vi "final.vi"() -> ()   [LabVIEW 2018]
uses:
  <vilib>/imath/engines/lvmath2/RunTimeEngine/Managers/WorkSpace/UID Generator.vi
  <vilib>/imath/engines/lvmath2/RunTimeEngine/RunTimeType/NIMS_RunTimeType_From StrictType (excl LVString).vi
  <instcachedir>/0/NIMS_RunTimeType_From StrictType (excl LVString)_E7E34A65C99947108168652BAD14964D.lvgen/NIMS_RunTimeType_From StrictType (excl LVString)_E7E34A65C99947108168652BAD14964D_000.vi
  <vilib>/imath/engines/lvmath2/RunTimeEngine/LocalVariableDefStatement/MC_LocalVariableDefStatement_Display.vi
  <vilib>/imath/engines/lvmath2/RunTimeEngine/RangeToken/NIMS_Range_R2 - Integer.vi
  <instcachedir>/0/NIMS_Range_R2 - Integer_E35B921DECF84AADB7325A02D418BFCC.lvgen/NIMS_Range_R2 - Integer_E35B921DECF84AADB7325A02D418BFCC_000.vi
  <vilib>/imath/engines/lvmath2/RunTimeEngine/CommandStatement/MC_CommandStatement_break.vi
  <vilib>/imath/engines/lvmath2/RunTimeEngine/IndexRead/NIMS V(S).vi
  <instcachedir>/0/NIMS V(S)_0488751826AF41519A22953C041130DC.lvgen/NIMS V(S)_0488751826AF41519A22953C041130DC_000.vi
  <vilib>/imathl/engines/lvmath/Functions/Error Handling/Create Error.vi
  <vilib>/imath/engines/lvmath2/RunTimeEngine/Managers/SymbolTable/Clear UID.vi
  <vilib>/imath/engines/lvmath2/RunTimeEngine/NodeEndStatement/NIMS_NodeEndStatement_Output.vi
  <instcachedir>/0/NIMS_NodeEndStatement_Output_53EC0D466D134D7ABD903AC30B43404B.lvgen/NIMS_NodeEndStatement_Output_53EC0D466D134D7ABD903AC30B43404B_011.vi
  <vilib>/imath/engines/lvmath2/RunTimeEngine/ErrorHandling/NIMS_Finalize Error.vi
  <vilib>/imath/engines/lvmath2/RunTimeEngine/BuiltInFunctions/acos/NIMS_acos(C).vi
  <instcachedir>/0/NIMS_acos(C)_EB9F8BBCD4F84158BAE4AC9B979C42E8.lvgen/NIMS_acos(C)_EB9F8BBCD4F84158BAE4AC9B979C42E8_001.vi
  <instcachedir>/0/NIMS_NodeEndStatement_Output_53EC0D466D134D7ABD903AC30B43404B.lvgen/NIMS_NodeEndStatement_Output_53EC0D466D134D7ABD903AC30B43404B_001.vi
  <vilib>/imath/engines/lvmath2/RunTimeEngine/Managers/SymbolTable/NIMS_WorkSpace.lvlib
panel:
  in  "Position 2":cluster{"X":dbl, "Y":dbl, "Theta":dbl}
  out "idx":i32=10
  in  "Position":cluster{"X":dbl, "Y":dbl, "Theta":dbl}
  out "range Out":dbl[](array[numeric])
  out "Position (mm)":cluster{"X":dbl, "Y":dbl, "Theta":dbl}
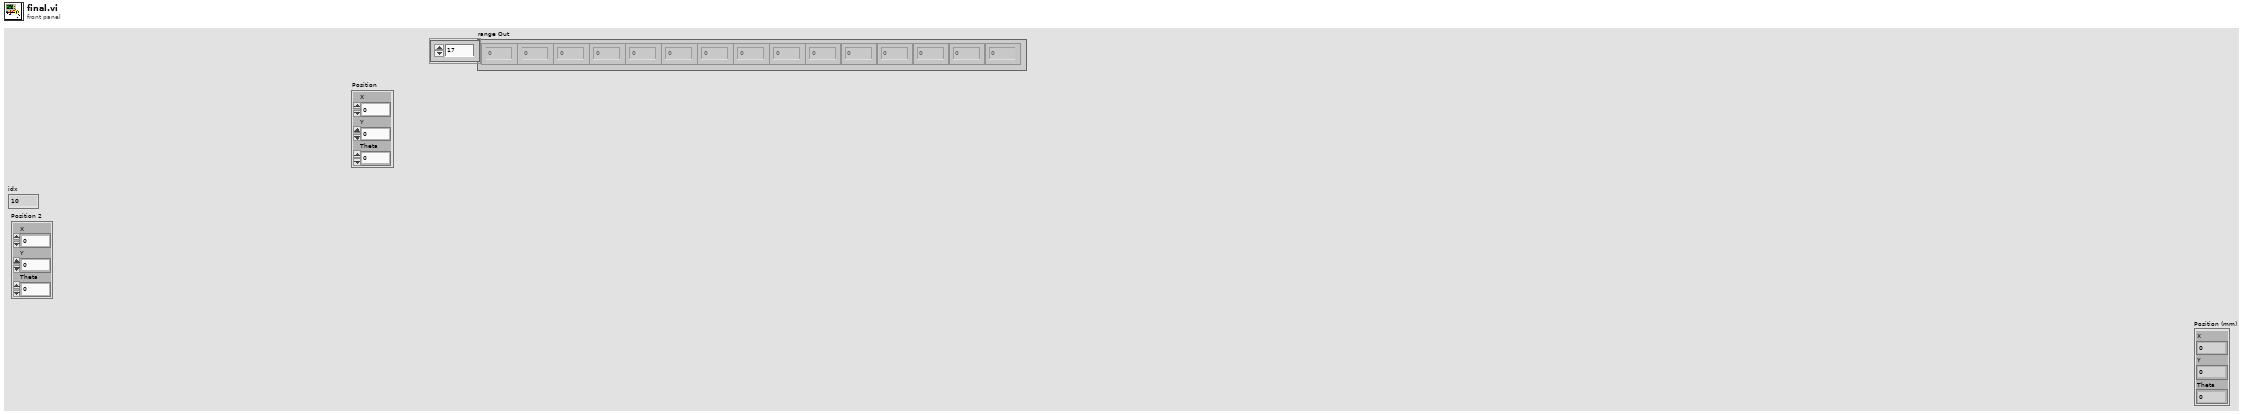
[diagram p1: front panel]
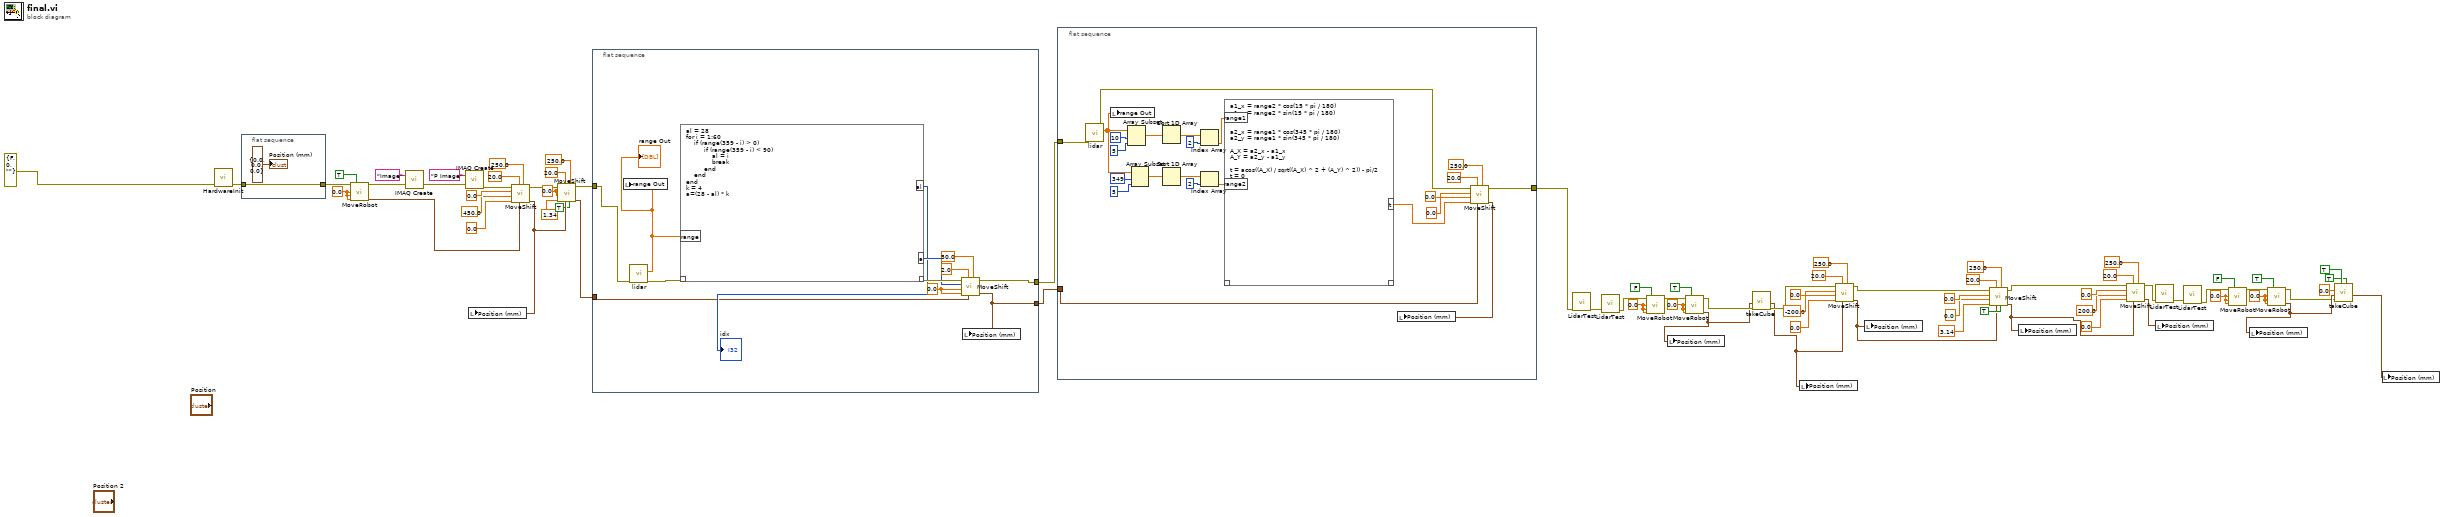
[diagram p0: block diagram]
diagram:
  w15 = 0.0 ("x (mm/s)")
  w12 = 0.0 ("x (mm/s)")
  w40 = 0.0 ("x (mm/s)")
  w43 = 0.0 ("x (mm/s)")
  w56 = 0.0 ("x shift")
  w74 = 0.0 ("x (mm/s)")
  n1 = call "HardwareInit.vi"("Error/Flow In"=errorcluster {"status"=FALSE, "code"=0, "source"=""}) -> ("error out"=w61:errorcluster)  [unwired: 10 in]
  n2 = flat-sequence {
    tunnel: w61 -> [w75]
    tunnel: [w75] -> w60
    frame #0 {
      "Position (mm)" <- cluster{"X":dbl, "Y":dbl, "Theta":dbl} {"X"=0.0, "Y"=0.0, "Theta"=0.0} ("Position (mm)")
    }
  }
  n3 = call "MoveRobot.vi"("Error/Flow In"=w60, "Reset"=TRUE, "x (mm/s)"=w74, "y (mm/s)"=w74, "theta (rad/s)"=w74) -> ("Error/Flow Out"=w72:errorcluster, "Position"=w62:cluster{"X":dbl, "Y":dbl, "Theta":dbl})  [unwired: 9 in]
  n4 = call "IMAQ Create"("Image Name"="Image", "error in (no error)"=w72) -> ("error out"=w70:errorcluster)  [unwired: 3 in, 1 out]
  n5 = call "IMAQ Create"("Image Name"="P Image", "error in (no error)"=w70) -> ("error out"=w68:errorcluster)  [unwired: 3 in, 1 out]
  n6 = call "MoveShift.vi"("max speed"=250.0, "Position"=w62, "Precision"=20.0, "theta"=0.0, "y shift"=450.0, "x shift"=0.0, "Error/Flow In"=w68) -> ("Position Out"=w57:cluster{"X":dbl, "Y":dbl, "Theta":dbl}, "Error/Flow Out"=w58:errorcluster)  [unwired: 3 in]
  n7 = local write "Position (mm)"(w57) -> ()
  n8 = call "MoveShift.vi"("UseTheta"=TRUE, "max speed"=250.0, "Position"=w57, "Precision"=20.0, "theta"=1.34, "y shift"=w56, "x shift"=w56, "Error/Flow In"=w58) -> ("Position Out"=w2:cluster{"X":dbl, "Y":dbl, "Theta":dbl}, "Error/Flow Out"=w4:errorcluster)  [unwired: 2 in]
  n9 = flat-sequence {
    tunnel: [w81] -> w5
    tunnel: [w80] -> w3
    tunnel: w4 -> [w79]
    tunnel: w2 -> [w78]
    frame #0 {
      w85 = 0.0 ("x shift")
      n10 = call "lidar.vi"("error in (no error)"=w79) -> ("error out"=w83:errorcluster, "range Out"=w77:dbl[])  [unwired: 8 in, 1 out]
      "range Out" <- w77
      n11 = local write "range Out"(w77) -> ()
      n12 = mathscript code="al = 28\nfor i = 1:60\n    if (range(359 - i) > 0)\n         if (range(359 - i) < 90)\n             al = i\n             break\n         end\n    end\nend\nk = 4\na=(28 - al) * k"("??"=w83, "range"=w77) -> ("??"=w88:errorcluster, "a"=w84:i32, "al"=→"idx":i32)
      n13 = call "MoveShift.vi"("max speed"=50.0, "Position"=w78, "Precision"=2.0, "theta"=w85, "y shift"=w85, "x shift"=w84, "Error/Flow In"=w88) -> ("Position Out"=w80:cluster{"X":dbl, "Y":dbl, "Theta":dbl}, "Error/Flow Out"=w81:errorcluster)  [unwired: 3 in]
      n14 = local write "Position (mm)"(w80) -> ()
    }
  }
  n15 = flat-sequence {
    tunnel: [w294] -> w1
    tunnel: w3 -> [w293]
    tunnel: w5 -> [w292]
    frame #0 {
      n16 = call "lidar.vi"("error in (no error)"=w292) -> ("error out"=w295:errorcluster, "range Out"=w309:dbl[])  [unwired: 8 in, 1 out]
      n17 = local write "range Out"(w309) -> ()
      n18 = Array Subset(array=w309, index=10, length=5) -> (w312:dbl[])
      n19 = Array Subset(array=w309, index=349, length=5) -> (w304:dbl[])
      n20 = Sort 1D Array(array=w312) -> (sorted array=w311:dbl[])
      n21 = Sort 1D Array(array=w304) -> (sorted array=w305:dbl[])
      n22 = Index Array(array=w311, index=2) -> (element=w303:dbl)
      n23 = Index Array(array=w305, index=2) -> (element=w302:dbl)
      n24 = mathscript code="a1_x = range2 * cos(15 * pi / 180)\na1_y = range2 * sin(15 * pi / 180)\n\n\na2_x = range1 * cos(345 * pi / 180)\na2_y = range1 * sin(345 * pi / 180)\n\nA_X = a2_x - a1_x\nA_Y = a2_y - a1_y\n\nt = acos((A_X) / sqrt((A_X) ^ 2 + (A_Y) ^ 2)) - pi/2\nt = 0"("range1"=w303, "range2"=w302) -> ("t"=w296:dbl)  [unwired: 1 in, 1 out]
      n25 = call "MoveShift.vi"("max speed"=250.0, "Position"=w293, "Precision"=20.0, "theta"=w296, "y shift"=0.0, "x shift"=0.0, "Error/Flow In"=w295) -> ("Position Out"=w301:cluster{"X":dbl, "Y":dbl, "Theta":dbl}, "Error/Flow Out"=w294:errorcluster)  [unwired: 3 in]
      n26 = local write "Position (mm)"(w301) -> ()
    }
  }
  n27 = call "LidarTest.vi"("error in"=w1) -> ("error out"=w51:errorcluster)  [unwired: 9 in]
  n28 = call "LidarTest.vi"("error in"=w51) -> ("error out"=w38:errorcluster)  [unwired: 9 in]
  n29 = call "MoveRobot.vi"("Error/Flow In"=w38, "Reset"=FALSE, "x (mm/s)"=w43, "y (mm/s)"=w43, "theta (rad/s)"=w43) -> ("Error/Flow Out"=w39:errorcluster)  [unwired: 9 in, 1 out]
  n30 = call "MoveRobot.vi"("Error/Flow In"=w39, "Reset"=TRUE, "x (mm/s)"=w40, "y (mm/s)"=w40, "theta (rad/s)"=w40) -> ("Error/Flow Out"=w37:errorcluster, "Position"=w36:cluster{"X":dbl, "Y":dbl, "Theta":dbl})  [unwired: 9 in]
  n31 = local write "Position (mm)"(w36) -> ()
  n32 = call "takeCube.vi"("Error/Flow In"=w37, "Position (mm)"=w36) -> ("error out"=w45:errorcluster, "Position Out"=w44:cluster{"X":dbl, "Y":dbl, "Theta":dbl})  [unwired: 8 in]
  n33 = local write "Position (mm)"(w44) -> ()
  n34 = call "MoveShift.vi"("max speed"=250.0, "Position"=w44, "Precision"=20.0, "theta"=0.0, "y shift"=-200.0, "x shift"=0.0, "Error/Flow In"=w45) -> ("Position Out"=w28:cluster{"X":dbl, "Y":dbl, "Theta":dbl}, "Error/Flow Out"=w30:errorcluster)  [unwired: 3 in]
  n35 = local write "Position (mm)"(w28) -> ()
  n36 = call "MoveShift.vi"("UseTheta"=TRUE, "max speed"=250.0, "Position"=w28, "Precision"=20.0, "theta"=3.14, "y shift"=0.0, "x shift"=0.0, "Error/Flow In"=w30) -> ("Position Out"=w21:cluster{"X":dbl, "Y":dbl, "Theta":dbl}, "Error/Flow Out"=w20:errorcluster)  [unwired: 2 in]
  n37 = local write "Position (mm)"(w21) -> ()
  n38 = call "MoveShift.vi"("max speed"=250.0, "Position"=w21, "Precision"=20.0, "theta"=0.0, "y shift"=200.0, "x shift"=0.0, "Error/Flow In"=w20) -> ("Position Out"=w27:cluster{"X":dbl, "Y":dbl, "Theta":dbl}, "Error/Flow Out"=w9:errorcluster)  [unwired: 3 in]
  n39 = call "LidarTest.vi"("error in"=w9) -> ("error out"=w10:errorcluster)  [unwired: 9 in]
  n40 = local write "Position (mm)"(w27) -> ()
  n41 = call "LidarTest.vi"("error in"=w10) -> ("error out"=w17:errorcluster)  [unwired: 9 in]
  n42 = call "MoveRobot.vi"("Error/Flow In"=w17, "Reset"=FALSE, "x (mm/s)"=w12, "y (mm/s)"=w12, "theta (rad/s)"=w12) -> ("Error/Flow Out"=w16:errorcluster)  [unwired: 9 in, 1 out]
  n43 = call "MoveRobot.vi"("Error/Flow In"=w16, "Reset"=TRUE, "x (mm/s)"=w15, "y (mm/s)"=w15, "theta (rad/s)"=w15) -> ("Error/Flow Out"=w18:errorcluster, "Position"=w19:cluster{"X":dbl, "Y":dbl, "Theta":dbl})  [unwired: 9 in]
  n44 = local write "Position (mm)"(w19) -> ()
  n45 = call "takeCube.vi"("ChangeCubes"=TRUE, "LeftArm"=TRUE, "Error/Flow In"=w18, "Position (mm)"=w19, "theta"=0.0) -> ("Position Out"=w11:cluster{"X":dbl, "Y":dbl, "Theta":dbl})  [unwired: 5 in, 1 out]
  n46 = local write "Position (mm)"(w11) -> ()
